vi "Local Mapper CTest.vi"(11 "GIC Input":T1={"     Use ?\nOff       On"=[FALSE, TRUE, FALSE, TRUE], "Mode:"=FALSE, "WP Data"="", "Hokuyo Port"="COM7", "Prop  Port"="COM6", "Compass Port"="", "GPS Port"="", "Num of WPs"=0, "WP Lats and Longs"={"WP Lats"=[], "WP Longs"=[]}, "Obst Lats and Longs"={"Obst Lats"=[], "Obst Longs"=[]}, "Parameters"=[], "GPS Data"=[], "Compass"=0.0, "LMS Vector"=[], "Vision Vector"=[], "Direction Cmd"=0.0, "Speed Cmd"=0.0, "WP Vector"=[], "WP Number"=0, "Extra"=0, "SW Map"=[], "Path Cluster"={"Path x node"=[], "Path y node"=[]}, "Sim Course"=[]} {"Obst Lats and Longs"."Obst Longs" format="%#_8g"; "Obst Lats and Longs"."Obst Lats" format="%#_8g"}) -> (3 "Local Map":picture)   [LabVIEW 2014]
panel:
  # "Local Mapper CTest"
  # "Input:"
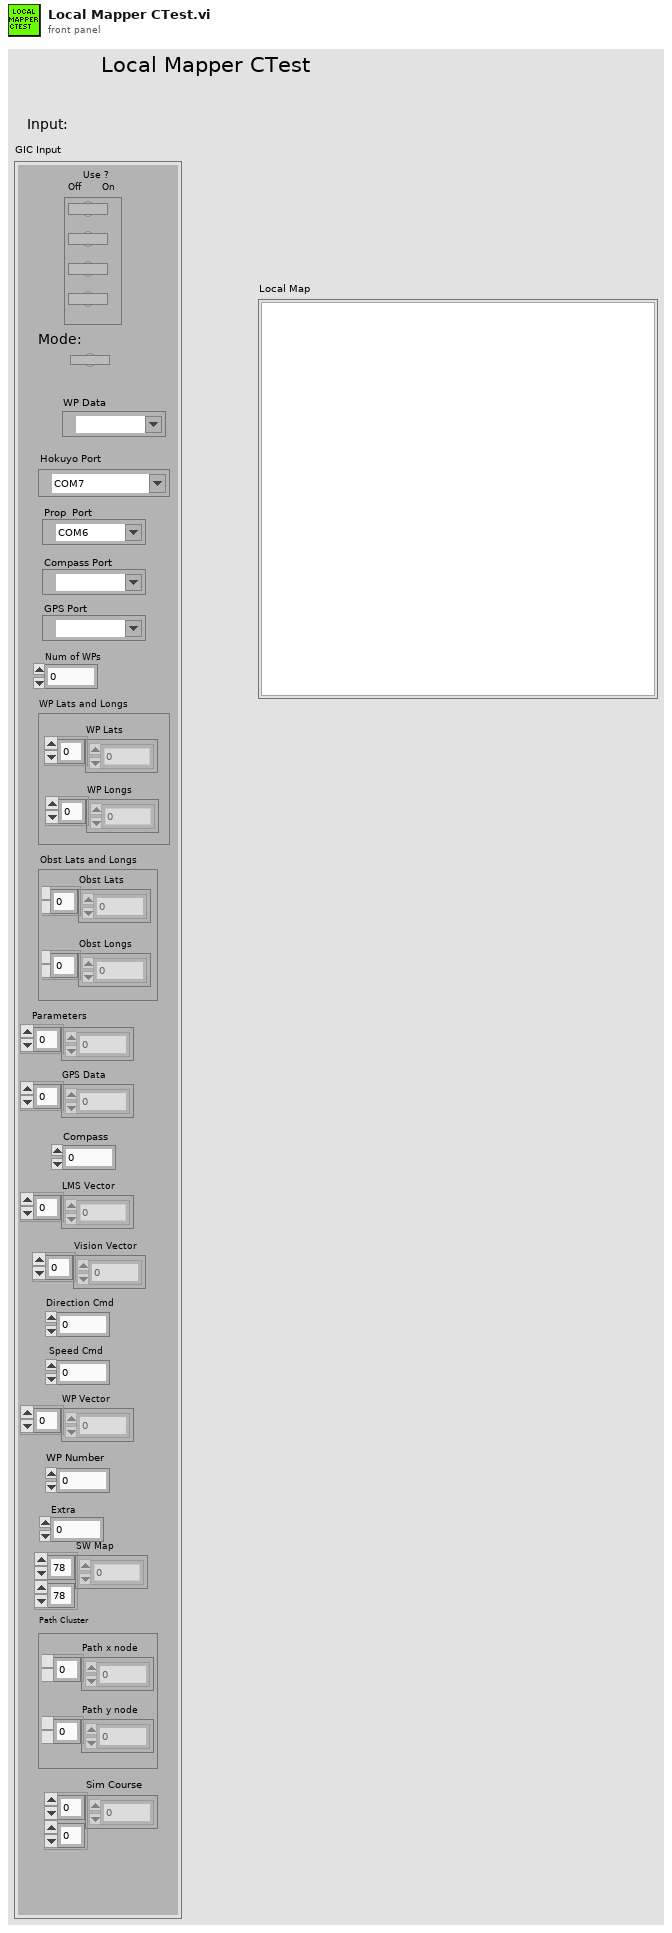
[diagram p1: front panel]
types:
  T1 = cluster{"     Use ?\nOff       On":bool[], "Mode:":bool, "WP Data":refnum<visa-resource-name>, "Hokuyo Port":refnum<visa-resource-name>, "Prop  Port":refnum<visa-resource-name>, "Compass Port":refnum<visa-resource-name>, "GPS Port":refnum<visa-resource-name>, "Num of WPs":i16, "WP Lats and Longs":cluster{"WP Lats":dbl[], "WP Longs":dbl[]}, "Obst Lats and Longs":cluster{"Obst Lats":dbl[], "Obst Longs":dbl[]}, "Parameters":dbl[], "GPS Data":dbl[], "Compass":dbl, "LMS Vector":dbl[], "Vision Vector":dbl[], "Direction Cmd":dbl, "Speed Cmd":dbl, "WP Vector":dbl[], "WP Number":i32, "Extra":i16, "SW Map":i32[][], "Path Cluster":cluster{"Path x node":dbl[], "Path y node":dbl[]}, "Sim Course":i8[][]}
  T2 = cluster{"Width":u16, "Style":enum32{"Solid", "Dash", "Dot", "DashDot", "DashDotDot"}}
  T3 = cluster{"left":i16, "top":i16, "right":i16, "bottom":i16}
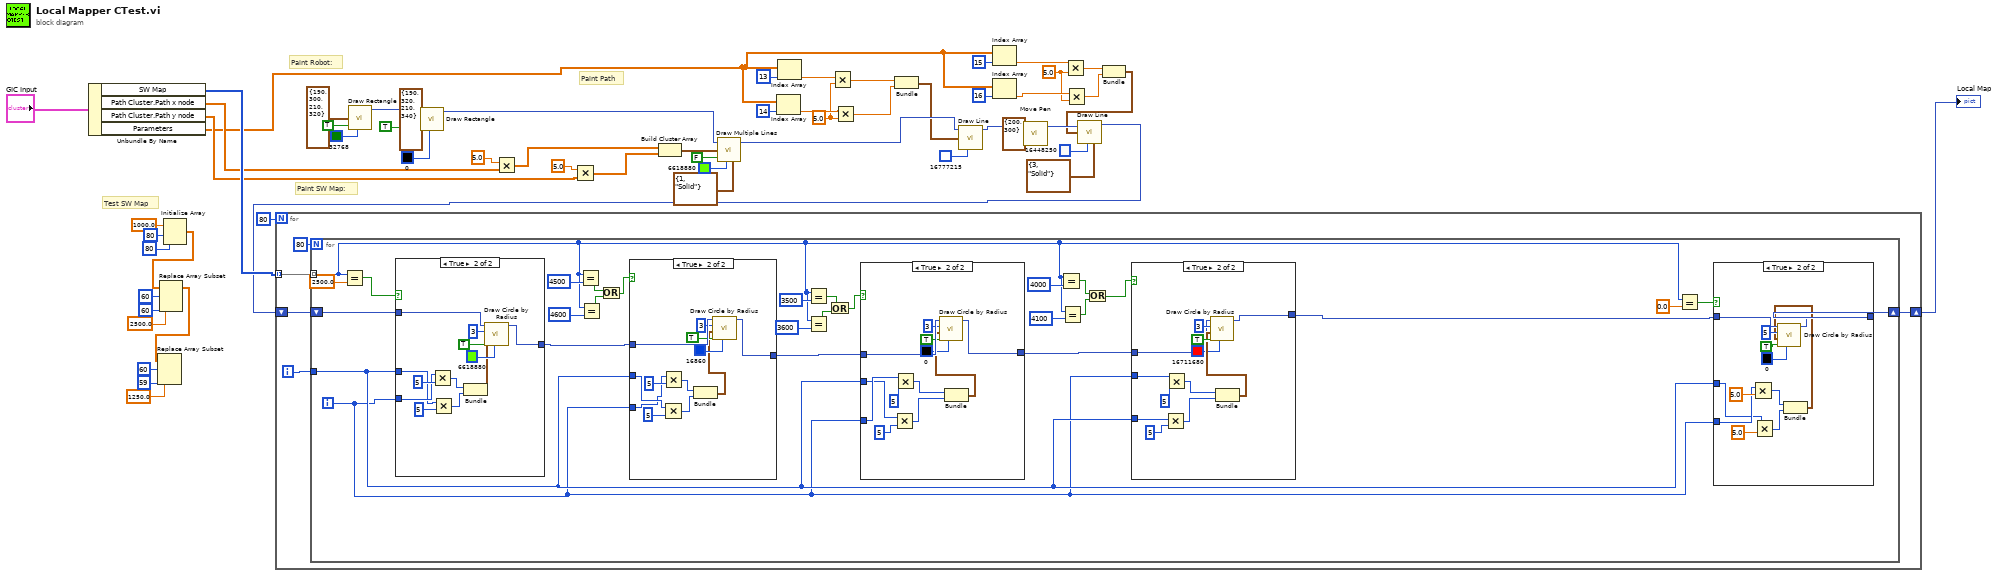
[diagram p0: block diagram]
diagram:
  w6 = 5.0 ("y")
  w19 = 5.0 ("y")
  # "Paint Path"
  # "Test SW Map"
  # "Paint SW Map:"
  # "Paint Robot:"
  n1 = Unbundle By Name("GIC Input") -> ("SW Map"=w38:i32[][], "Path Cluster.Path x node"=w36:dbl[], "Path Cluster.Path y node"=w34:dbl[], "Parameters"=w12:dbl[])
  n2 = Initialize Array(1000.0 ("element"), 80 ("dimension size"), 80 ("dimension size")) -> (w48:dbl[][])
  n3 = Replace Array Subset(array=w48, new element=2500.0 ("new element/subarray"), index (row)=60, index (col)=60 ("disabled index (col)")) -> (w42:dbl[][])
  n4 = Replace Array Subset(array=w42, new element=1250.0 ("new element/subarray"), index (row)=60, index (col)=59 ("disabled index (col)")) -> ()  [unwired: 1 out]
  n5 = call <vilib>:"Draw Rectangle.vi"("rect"=T3 {"left"=190, "top"=300, "right"=210, "bottom"=320}, "fill?(F)"=TRUE, "color(black)"=u32 32768) -> ("new picture"=w55:picture)  [unwired: 6 in]
  n6 = call <vilib>:"Draw Rectangle.vi"("picture"=w55, "rect"=T3 {"left"=190, "top"=320, "right"=210, "bottom"=340}, "fill?(F)"=TRUE, "color(black)"=u32 0) -> ("new picture"=w27:picture)  [unwired: 5 in]
  n7 = Multiply(x=5.0, y=w36) -> (x*y=w33:dbl[])
  n8 = Multiply(x=5.0, y=w34) -> (x*y=w32:dbl[])
  n9 = Build Cluster Array(w33, w32) -> (w31:cluster{dbl, dbl}[])
  n10 = call <vilib>:"Draw Multiple Lines.vi"("picture"=w27, "line endpoints"=w31, "fill?(F)"=FALSE, "color(black)"=u32 6618880, "pen"=T2 {"Width"=1, "Style"=enum."Solid"}) -> ("new picture"=w26:picture)  [unwired: 4 in]
  n11 = Index Array(array=w12, index=14) -> (element=w21:dbl)
  n12 = Index Array(array=w12, index=13) -> (element=w18:dbl)
  n13 = Multiply(x=w18, y=w19) -> (x*y=w17:dbl)
  n14 = Multiply(x=w21, y=w19) -> (x*y=w20:dbl)
  n15 = Bundle(w17, w20) -> (w22:cluster{dbl, dbl})  [unwired: 1 in]
  n16 = call <vilib>:"Draw Line.vi"("picture"=w26, "end point"=w22, "color(black)"=u32 16777215) -> ("new picture"=w14:picture)  [unwired: 6 in]
  n17 = Index Array(array=w12, index=15) -> (element=w8:dbl)
  n18 = Index Array(array=w12, index=16) -> (element=w7:dbl)
  n19 = call <vilib>:"Move Pen.vi"("new position"=cluster{"x":i16, "y":i16} {"x"=200, "y"=300}, "picture"=w14) -> ("new picture"=w15:picture)  [unwired: 3 in]
  n20 = Multiply(x=w8, y=w6) -> (x*y=w9:dbl)
  n21 = Multiply(x=w7, y=w6) -> (x*y=w5:dbl)
  n22 = Bundle(w9, w5) -> (w4:cluster{dbl, dbl})  [unwired: 1 in]
  n23 = call <vilib>:"Draw Line.vi"("picture"=w15, "end point"=w4, "color(black)"=u32 16448250, "pen"=T2 {"Width"=3, "Style"=enum."Solid"}) -> ("new picture"=w16:picture)  [unwired: 5 in]
  n24 = for {
    N: 80 -> [_]
    tunnel: w38 -> [w62] mode=indexing
    shift-right: [w60] -> w44
    shift-left: w16 -> [w61]
    i -> [w59]
    n25 = for {
      N: 80 -> [_]
      tunnel: w62 -> [w65] mode=indexing
      shift-right: [w86] -> w60
      shift-left: w61 -> [w89]
      tunnel: w59 -> [w67]
      i -> [w66]
      n26 = Equal?(x=w65, y=2500.0) -> (x = y?=w90:bool)
      n27 = case shown="True" w90 {
        tunnel: w89 -> [w144 w153]
        tunnel: [w144 w150] -> w87
        tunnel: w66 -> [_ w146]
        tunnel: w67 -> [_ w145]
        frame False {
        }
        frame True {
          n28 = Multiply(x=w146, y=5) -> (x*y=w149:i32)
          n29 = Multiply(x=w145, y=5) -> (x*y=w148:i32)
          n30 = Bundle(w149, w148) -> (w147:cluster{i32, i32})  [unwired: 1 in]
          n31 = call <vilib>:"Draw Circle by Radius.vi"("color(black)"=u32 6618880, "fill?(F)"=TRUE, "pixel center"=w147, "radius"=i16 3, "picture"=w153) -> ("new picture"=w150:picture)  [unwired: 6 in]
        }
      }
      n32 = Equal?(x=w65, y=4500) -> (x = y?=w78:bool)
      n33 = Equal?(x=w65, y=4600) -> (x = y?=w77:bool)
      n34 = Or(x=w78, y=w77) -> (x .or. y?=w76:bool)
      n35 = case shown="True" w76 {
        tunnel: w87 -> [w131 w143]
        tunnel: [w131 w142] -> w83
        tunnel: w67 -> [_ w133]
        tunnel: w66 -> [_ w132]
        frame False {
        }
        frame True {
          n36 = Multiply(x=w133, y=5) -> (x*y=w135:i32)
          n37 = Multiply(x=w132, y=5) -> (x*y=w136:i32)
          n38 = Bundle(w136, w135) -> (w134:cluster{i32, i32})  [unwired: 1 in]
          n39 = call <vilib>:"Draw Circle by Radius.vi"("color(black)"=u32 16860, "fill?(F)"=TRUE, "pixel center"=w134, "radius"=i16 3, "picture"=w143) -> ("new picture"=w142:picture)  [unwired: 6 in]
        }
      }
      n40 = Equal?(x=w65, y=3500) -> (x = y?=w70:bool)
      n41 = Equal?(x=w65, y=3600) -> (x = y?=w69:bool)
      n42 = Or(x=w70, y=w69) -> (x .or. y?=w68:bool)
      n43 = case shown="True" w68 {
        tunnel: w83 -> [w105 w117]
        tunnel: [w105 w107] -> w80
        tunnel: w67 -> [_ w111]
        tunnel: w66 -> [_ w112]
        frame False {
        }
        frame True {
          n44 = Multiply(x=w111, y=5) -> (x*y=w114:i32)
          n45 = Multiply(x=w112, y=5) -> (x*y=w113:i32)
          n46 = Bundle(w113, w114) -> (w108:cluster{i32, i32})  [unwired: 1 in]
          n47 = call <vilib>:"Draw Circle by Radius.vi"("color(black)"=u32 0, "fill?(F)"=TRUE, "pixel center"=w108, "radius"=i16 3, "picture"=w117) -> ("new picture"=w107:picture)  [unwired: 6 in]
        }
      }
      n48 = Equal?(x=w65, y=4000) -> (x = y?=w74:bool)
      n49 = Equal?(x=w65, y=4100) -> (x = y?=w73:bool)
      n50 = Or(x=w74, y=w73) -> (x .or. y?=w72:bool)
      n51 = case shown="True" w72 {
        tunnel: [w92 w97] -> w64
        tunnel: w80 -> [w92 w95]
        tunnel: w67 -> [_ w93]
        tunnel: w66 -> [_ w94]
        frame False {
        }
        frame True {
          n52 = Multiply(x=w93, y=5) -> (x*y=w102:i32)
          n53 = Multiply(x=w94, y=5) -> (x*y=w101:i32)
          n54 = Bundle(w101, w102) -> (w98:cluster{i32, i32})  [unwired: 1 in]
          n55 = call <vilib>:"Draw Circle by Radius.vi"("color(black)"=u32 16711680, "fill?(F)"=TRUE, "pixel center"=w98, "radius"=i16 3, "picture"=w95) -> ("new picture"=w97:picture)  [unwired: 6 in]
        }
      }
      n56 = Equal?(x=w65, y=0.0) -> (x = y?=w85:bool)
      n57 = case shown="True" w85 {
        tunnel: w64 -> [w118 w130]
        tunnel: [w118 w129] -> w86
        tunnel: w67 -> [_ w120]
        tunnel: w66 -> [_ w121]
        frame False {
        }
        frame True {
          n58 = Multiply(x=w121, y=5.0) -> (x*y=w124:i32)
          n59 = Multiply(x=w120, y=5.0) -> (x*y=w123:i32)
          n60 = Bundle(w124, w123) -> (w122:cluster{i32, i32})  [unwired: 1 in]
          n61 = call <vilib>:"Draw Circle by Radius.vi"("color(black)"=u32 0, "fill?(F)"=TRUE, "pixel center"=w122, "radius"=i16 5, "picture"=w130) -> ("new picture"=w129:picture)  [unwired: 6 in]
        }
      }
    }
  }
  "Local Map" <- w44
